vi "List Available Cylinders for Knock Sensor.vi"(8 "error in (no error)":errorcluster, 10 "Timing measurement":string, 11 "Item Ref in":T1 format="%.0x") -> (0 "error out":errorcluster, 2 "cylinders available":string[](array[string]), 3 "Item Ref out":T1 format="%.0x")   [LabVIEW 2013, in "Engine Simulation Toolkit System Explorer.lvlib"]
uses:
  Engine Simulation Toolkit System Explorer.lvlib
  <vilib>/NI Veristand/Custom Device API/Custom Device Item Ref.ctl
  Shared/Properties.vi
  Shared/Engine Simulation Toolkit Shared.lvlib
  <vilib>/NI Veristand/Custom Device API/Custom Device API.lvlib
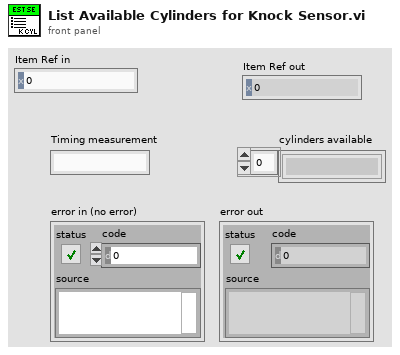
[diagram p1: front panel]
types:
  T1 = typedef "Custom Device API.lvlib/Custom Device Item Ref.ctl" = u64
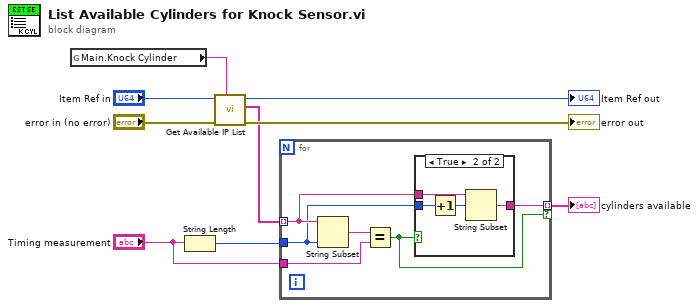
[diagram p0: block diagram]
diagram:
  n1 = global read "Properties.vi" "Main.Knock Cylinder"() -> (w5:string)
  n2 = String Length(string="Timing measurement") -> (length=w3:i32)
  n3 = call "Get Available IP List.vi"("ip list property name"=w5, "error in (no error)"="error in (no error)", "Item Ref in"="Item Ref in") -> ("error out"=→"error out":errorcluster, "ips available"=w4:string[], "Item Ref out"=→"Item Ref out":T1)  [unwired: 6 in]
  n4 = for {
    tunnel: w4 -> [w13] mode=indexing
    tunnel: w3 -> [w12]
    tunnel: "Timing measurement" -> [w14]
    tunnel: [w11] -> w1 mode=indexing if=w10
    n5 = String Subset(string=w13, length (rest)=w12) -> (substring=w15:string)  [unwired: 1 in]
    n6 = Equal?(x=w15, y=w14) -> (x = y?=w10:bool)
    n7 = case shown="True" w10 {
      tunnel: w13 -> [_ w19]
      tunnel: w12 -> [_ w17]
      tunnel: [_ w18] -> w11
      frame False {
      }
      frame True {
        n8 = Increment(x=w17) -> (x+1=w16:i32)
        n9 = String Subset(string=w19, offset (0)=w16) -> (substring=w18:string)  [unwired: 1 in]
      }
    }
  }
  "cylinders available" <- w1
